vi "Thorlabs_CageRotator_ActiveX.vi"(8 "error in (no error)":errorcluster, 11 "HWSerialNum":i32=27264338) -> (0 "error out":errorcluster)   [LabVIEW 2022 SP3]
panel:
  in  "stop":bool
  in  "MG17Motor":refnum<k7>(container)
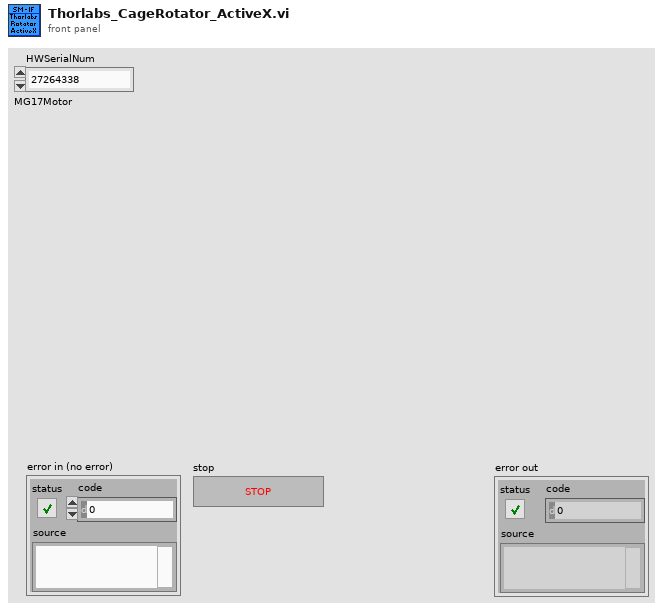
[diagram p1: front panel]
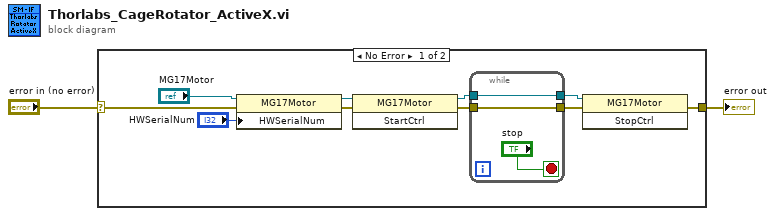
[diagram p0: block diagram]
diagram:
  n1 = case shown="No Error" "error in (no error)" {
    selector: "error in (no error)" -> [w3 w16]
    tunnel: [w4 w16] -> w2
    frame No Error {
      n2 = property class="MG17Motor"(reference="MG17Motor", error in=w3, "HWSerialNum"="HWSerialNum") -> (reference out=w10:refnum<k7>, error out=w9:errorcluster)
      n3 = invoke class="MG17Motor" method="StartCtrl"(reference=w10, error in=w9) -> (reference out=w7:refnum<k7>, error out=w5:errorcluster)  [unwired: 1 in, 1 out]
      n4 = while {
        tunnel: [w15] -> w8
        tunnel: w7 -> [w15]
        tunnel: [w14] -> w6
        tunnel: w5 -> [w14]
        stop <- "stop" stop-if-true
      }
      n5 = invoke class="MG17Motor" method="StopCtrl"(reference=w8, error in=w6) -> (error out=w4:errorcluster)  [unwired: 1 in, 2 out]
    }
    frame Error {
    }
  }
  "error out" <- w2
